vi "SetLabel.vi"(8 "error in (no error)":errorcluster caption="错误输入（无错误）", 11 "XYPlot 输入":refnum<class "XYPlot.lvclass">) -> (0 "error out":errorcluster caption="错误输出", 3 "XYPlot 输出":refnum<class "XYPlot.lvclass">)   [LabVIEW 2018, in "DataDisplay.lvlib" / "XYPlot.lvclass"]
uses:
  XYPlot.lvclass
  XYPlot.lvclass/XYPlot.ctl
  SubVI/DD_Parameter.vi
  DataDisplay.lvlib
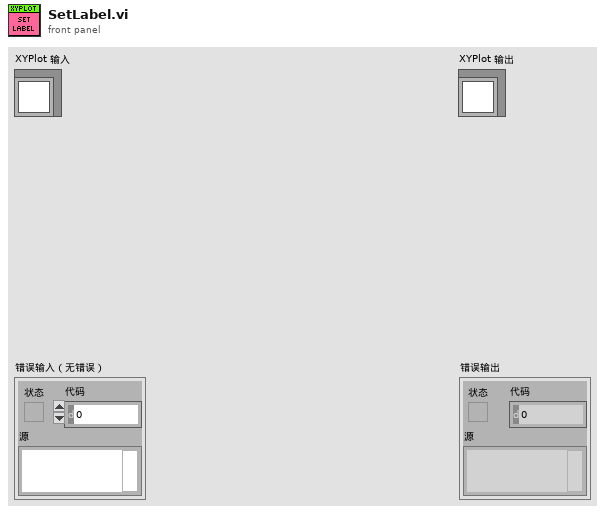
[diagram p1: front panel]
types:
  T1 = typedef "DataDisplay.lvlib/DD_ChannelInfo.ctl" = cluster{"名称":string, "单位":string, "数据类型":enum16{"Real", "Int"}, "趋势线":enum16{"N/A", "X", "Y"}}
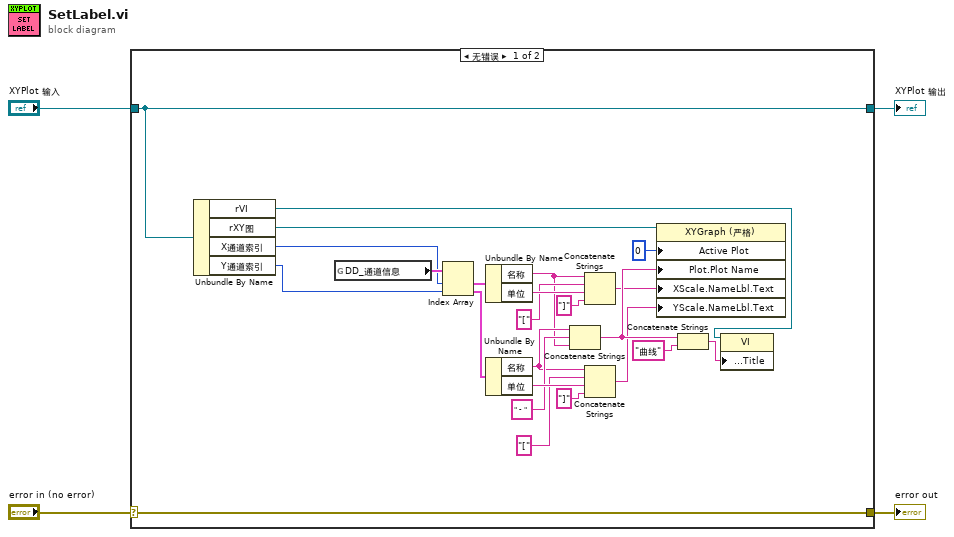
[diagram p0: block diagram]
diagram:
  n1 = case shown="无错误" "error in (no error)" {
    selector: "error in (no error)" -> [w28 w30]
    tunnel: [w28 w30] -> w3
    tunnel: [w27 w29] -> w1
    tunnel: "XYPlot 输入" -> [w27 w29]
    frame No Error {
      n2 = Unbundle By Name(w27) -> ("rVI"=w11:refnum<vi>, "rXY图"=w10:refnum<vi>, "X通道索引"=w8:i32, "Y通道索引"=w7:i32)
      n3 = global read "DD_Parameter.vi" "DD_通道信息"() -> (w9:T1[])
      n4 = Index Array(array=w9, index #1=w8, index #2=w7) -> (element #1=w20:T1, element #2=w21:T1)
      n5 = Unbundle By Name(w20) -> ("名称"=w5:string, "单位"=w22:string)
      n6 = Unbundle By Name(w21) -> ("名称"=w6:string, "单位"=w24:string)
      n7 = Concatenate Strings(w6, " - " ("字符串"), w5) -> (w26:string)
      n8 = Concatenate Strings(w5, "[" ("字符串"), w22, "]" ("字符串")) -> (w23:string)
      n9 = Concatenate Strings(w6, "[" ("字符串"), w24, "]" ("字符串")) -> (w25:string)
      n10 = property class="XYGraph (严格)"(reference=w10, "Active Plot"=u32 0 ("活动曲线"), "Plot.Plot Name"=w26, "XScale.NameLbl.Text"=w23, "YScale.NameLbl.Text"=w25) -> ()  [unwired: 1 in, 2 out]
      n11 = Concatenate Strings(w26, "曲线" ("字符串")) -> (w19:string)
      n12 = property class="VI"(reference=w11, "Front Panel.Title"=w19) -> ()  [unwired: 1 in, 2 out]
    }
    frame Error {
    }
  }
  "error out" <- w3
  "XYPlot 输出" <- w1
